vi "Optionen_Setzen_Sicherungskopie.vi"(8 "error in (no error)":errorcluster caption="Fehler (Eingang, kein Fehler)", 10 "Optionen (Eingang)":T1 {"SP laden speichern" items=["SP1"=1, "SP2"=2]; "Span Gas Auswahl" items=["1"=1, "2"=2, "3"=3, "4"=4, "5"=5, "6"=6, "7"=7, "8"=8]}, 11 "Cluster (Eingang)":refnum<vi>) -> (0 "error out":errorcluster caption="Fehler (Ausgang)")   [LabVIEW 2020]
uses:
  System Einstellungen/Optionen.ctl
  Funktionstasten/Spaneingang.ctl
  Funktionstasten/Funktionstasten.lvlib
  System Einstellungen/System Einstellungen.lvlib
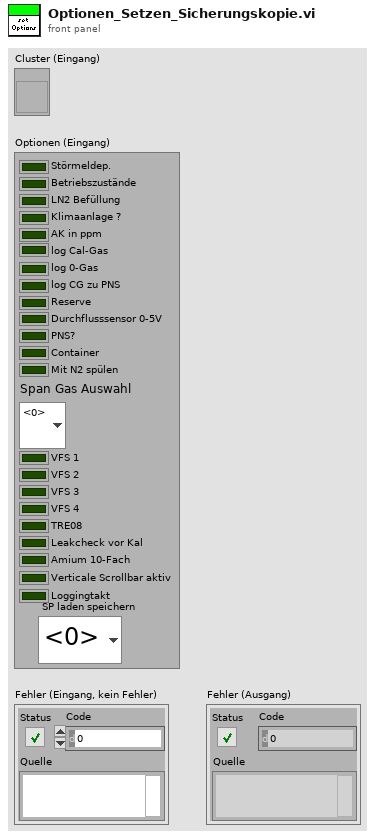
[diagram p1: front panel]
types:
  T1 = typedef "System Einstellungen.lvlib/Optionen.ctl" = cluster{"Störmeldep.":bool, "Betriebszustände":bool, "LN2 Befüllung":bool, "Klimaanlage ?":bool, "AK in ppm":bool, "log Cal-Gas":bool, "log 0-Gas":bool, "log CG zu PNS":bool, "Reserve":bool, "Durchflusssensor 0-5V":bool, "PNS?":bool, "Container":bool, "Mit N2 spülen":bool, "Span Gas Auswahl":T2, "VFS 1":bool, "VFS 2":bool, "VFS 3":bool, "VFS 4":bool, "TRE08":bool, "Leakcheck vor Kal":bool, "Amium 10-Fach":bool, "Verticale Scrollbar aktiv":bool, "Loggingtakt":bool, "SP laden speichern":u16}
  T2 = typedef "Funktionstasten.lvlib/Spaneingang.ctl" = u16
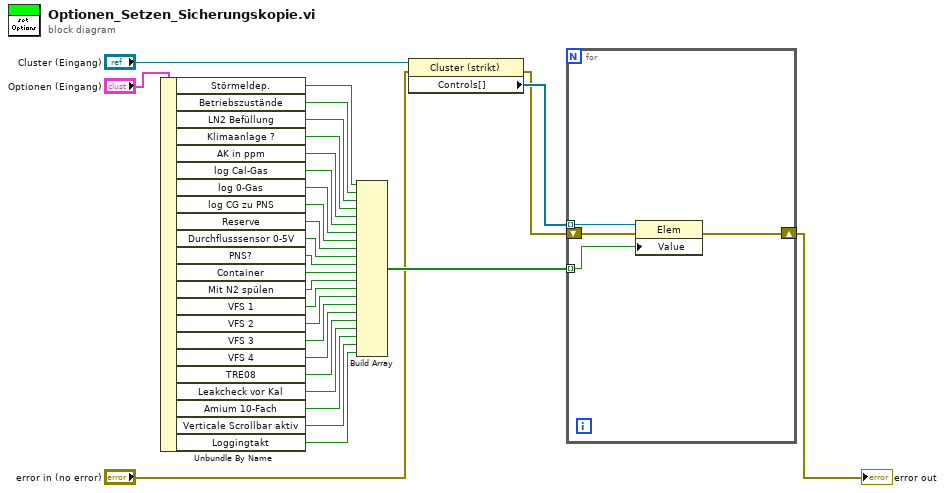
[diagram p0: block diagram]
diagram:
  n1 = Unbundle By Name("Optionen (Eingang)") -> ("Störmeldep."=w28:bool, "Betriebszustände"=w27:bool, "LN2 Befüllung"=w26:bool, "Klimaanlage ?"=w25:bool, "AK in ppm"=w24:bool, "log Cal-Gas"=w23:bool, "log 0-Gas"=w22:bool, "log CG zu PNS"=w21:bool, "Reserve"=w20:bool, "Durchflusssensor 0-5V"=w19:bool, "PNS?"=w18:bool, "Container"=w17:bool, "Mit N2 spülen"=w16:bool, "VFS 1"=w15:bool, "VFS 2"=w14:bool, "VFS 3"=w13:bool, "VFS 4"=w12:bool, "TRE08"=w11:bool, "Leakcheck vor Kal"=w10:bool, "Amium 10-Fach"=w9:bool, "Verticale Scrollbar aktiv"=w8:bool, "Loggingtakt"=w7:bool)
  n2 = Build Array(w28, w27, w26, w25, w24, w23, w22, w21, w20, w19, w18, w17, w16, w15, w14, w13, w12, w11, w10, w9, w8, w7) -> (w4:bool[])
  n3 = property class="Cluster (strikt)"(reference="Cluster (Eingang)", error in="error in (no error)") -> (error out=w3:errorcluster, "Controls[]"=w5:refnum<vi>[])  [unwired: 1 out]
  n4 = for {
    tunnel: w5 -> [w33] mode=indexing
    tunnel: w4 -> [w32] mode=indexing
    shift-right: [w30] -> w2
    shift-left: w3 -> [w31]
    n5 = property class="Elem"(reference=w33, error in=w31, "Value"=w32) -> (error out=w30:errorcluster)  [unwired: 1 out]
  }
  "error out" <- w2
